vi "optoNCDT_A_in.vi"() -> ()   [LabVIEW 2026]
uses:
  <vilib>/DAQmx/read.llb/DAQmx Read.vi
  <vilib>/DAQmx/read.llb/DAQmx Read (Analog 1D Wfm NChan NSamp).vi
  <vilib>/DAQmx/miscellaneous.llb/DAQmx Fill In Error Info.vi
panel:
  out "mm":dbl
  in  "stop":bool
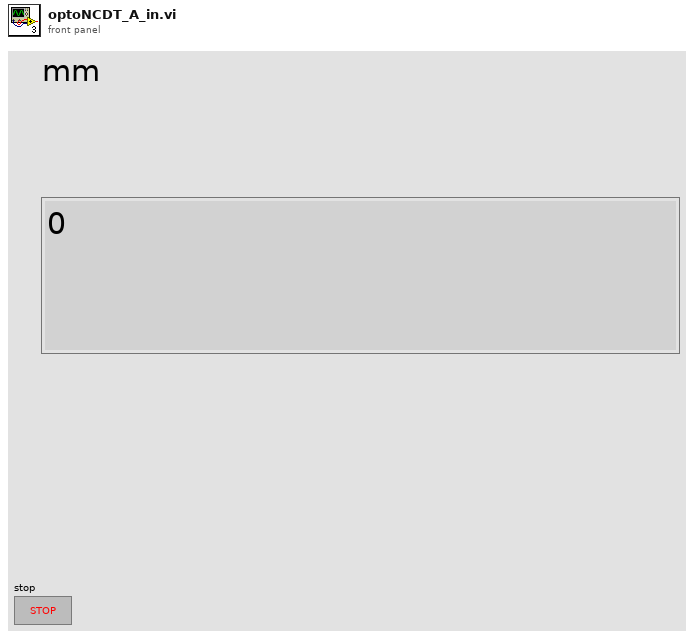
[diagram p1: front panel]
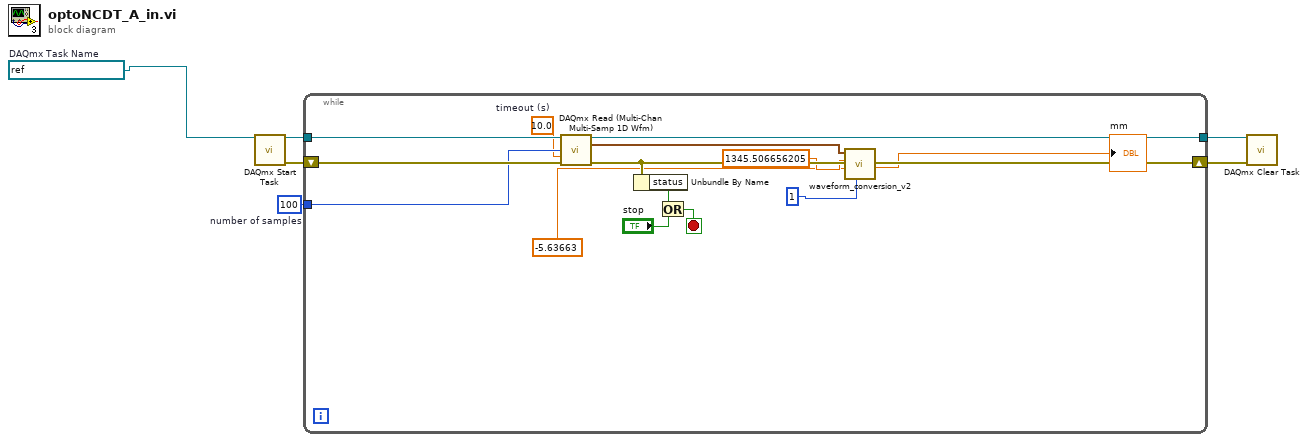
[diagram p0: block diagram]
diagram:
  w1 = refnum<k21> "optoNCDTsignal"  # DAQmx Task Name
  w4 = 100  # number of samples
  n1 = call <vilib>:"DAQmx Start Task.vi"("task/channels in"=w1) -> ("task out"=w6:refnum<k21>, "error out"=w5:errorcluster)  [unwired: 13 in]
  n2 = while {
    tunnel: w6 -> [w20]
    tunnel: w4 -> [w17]
    tunnel: [w18] -> w2
    shift-right: [w15] -> w3
    shift-left: w5 -> [w19]
    stop <- w14 stop-if-true
    w12 = 10.0  # timeout (s)
    n3 = call-poly "DAQmx Read (Multi-Chan Multi-Samp 1D Wfm).vi"("task/channels in"=w20, "number of samples per channel"=w17, "timeout"=w12, "error in"=w19) -> ("task out"=w18:refnum<k21>, "data"=w9:waveform(dbl)[], "error out"=w15:errorcluster)  [unwired: 9 in]
    n4 = Unbundle By Name(w15) -> ("status"=w16:bool)
    n5 = Or(x=w16, y="stop") -> (x .or. y?=w14:bool)
    n6 = call "waveform_conversion_v2.vi"("sample length"=1, "y"=-5.63663, "y 2"=1345.506656205 ("y"), "data"=w9) -> ("mean"=→"mm":dbl)  [unwired: 7 in]
  }
  n7 = call <vilib>:"DAQmx Clear Task.vi"("task in"=w2, "error in"=w3) -> ()  [unwired: 13 in, 1 out]
